vi "Ture to Flase.vi"(5 "in":bool) -> (2 "Out":bool)   [LabVIEW 2014]
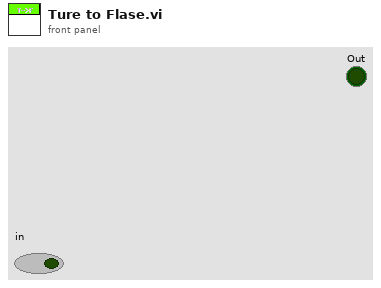
[diagram p1: front panel]
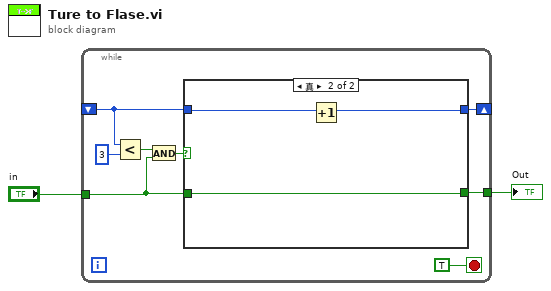
[diagram p0: block diagram]
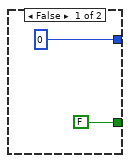
[diagram p2: hidden frame]
diagram:
  n1 = while {
    shift-right: [w7] -> _
    shift-left: _ -> [w8]
    tunnel: "in" -> [w4]
    tunnel: [w3] -> w1
    stop <- TRUE stop-if-true
    n2 = Less?(x=w8, y=3) -> (x < y?=w5:bool)
    n3 = And(x=w5, y=w4) -> (x .and. y?=w6:bool)
    n4 = case shown="真" w6 {
      tunnel: w8 -> [_ w15]
      tunnel: [0 w14] -> w7
      tunnel: w4 -> [_ w13]
      tunnel: [FALSE w13] -> w3
      frame False {
      }
      frame True {
        n5 = Increment(x=w15) -> (x+1=w14:i32)
      }
    }
  }
  "Out" <- w1
